vi "Set Kernel Arguments Memory Object.vi"(8 "Error In":errorcluster, 9 "Kernel Handle":T6, 10 "Argument Number":i32, 11 "Memory Object":T1 {"Dimension"."Width" min=1; "Dimension"."Height" min=1; "Dimension"."Depth" min=1}) -> (0 "Error Out":errorcluster, 1 "Kernel Handle out":T6, 2 "Auto Inc Arugment Number":i32)   [LabVIEW 2012, in "OpenCLV x64.lvlib"]
doc: "Sets an argument of a kernel to a device memory object. This must be used with any kernel call that is __global, regardless of the type of memory used in the kernel.\n\nFor example, __global float *Data_32f and __global double *Data_64f would both be set using this VI."
uses:
  OpenCLV x64.lvlib
  Controls/Kernel Handle.ctl
  Controls/Memory Object.ctl
  Controls/Device ID.ctl
  Controls/Memory ID.ctl
  User Controls/Array Dimensions.ctl
  Controls/Memory Type.ctl
  Error Checking/Add Error Functional Global.vi
panel:
  in  "Local Data?":bool
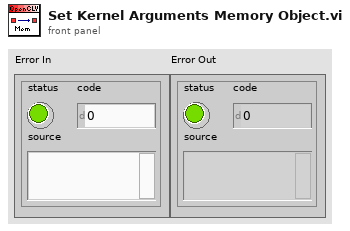
[diagram p1: front panel]
types:
  T1 = typedef "OpenCLV x64.lvlib/Memory Object.ctl" = cluster{"Device ID":T2, "Memeroy ID":T3, "Dimension":T4, "Memory Type":T5}
  T2 = typedef "OpenCLV x64.lvlib/Device ID.ctl" = u64
  T3 = typedef "OpenCLV x64.lvlib/Memory ID.ctl" = u64
  T4 = typedef "Array Dimensions.ctl" = cluster{"Depth":u64, "Height":u64, "Width":u64}
  T5 = typedef "OpenCLV x64.lvlib/Memory Type.ctl" = enum16{"32f", "u8", "i8", "u16", "i16", "u32", "i32", "64f"}
  T6 = typedef "OpenCLV x64.lvlib/Kernel Handle.ctl" = u64
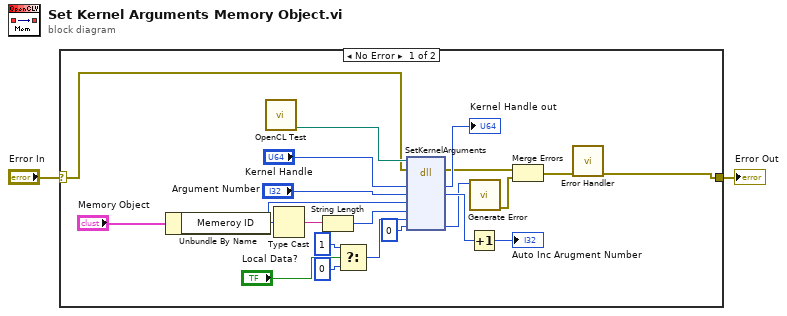
[diagram p0: block diagram]
diagram:
  n1 = case shown="No Error" "Error In" {
    selector: "Error In" -> [w3 w24]
    tunnel: [w7 w24] -> w1
    frame No Error {
      n2 = Unbundle By Name("Memory Object") -> ("Memeroy ID"=w13:T3)
      n3 = call "OpenCL Test.vi"() -> ("DLL To Use"=w8:path)  [unwired: 11 in]
      n4 = Type Cast(x=w13) -> (*(type *) &x=w16:string)  [unwired: 1 in]
      n5 = String Length(string=w16) -> (length=w15:i32)
      n6 = Select(t=1, s="Local Data?", f=0 ("t")) -> (s? t:f=w9:i32)
      n7 = dll-call lib="C:/Users/bme-amcelroy-la/Desktop/OpenCLV/trunk/OpenCLV_x64_1.0/OpenCLV_x64.dll" fn="SetKernelArguments"(path in=w8, error in=w3, "Kernel Handle"="Kernel Handle", "Argument Number"="Argument Number", "Data"=w13, "Size of Data Pointer in bytes"=w15, "Local"=w9, "Error"=0) -> (error out=w5:errorcluster, "Kernel Handle"=→"Kernel Handle out":u64, "Argument Number"=w19:i32, "Error"=w17:i32)  [unwired: 5 in, 1 out]
      n8 = Increment(x=w19) -> (x+1=→"Auto Inc Arugment Number":i32)
      n9 = call "Generate Error.vi"("Error"=w17) -> ("error out"=w6:errorcluster)  [unwired: 10 in]
      n10 = Merge Errors(w5, w6) -> (w4:errorcluster)
      n11 = call-poly "Error Handler.vi"("Error In"=w4) -> ("Error Out"=w7:errorcluster)  [unwired: 10 in]
    }
    frame Error {
    }
  }
  "Error Out" <- w1
